vi "Get Table Configuration.vi"(8 "error in (no error)":errorcluster, 11 "Basic Table in":refnum<class "Basic Table.lvclass">) -> (0 "error out":errorcluster, 2 "Table Configuration":refnum<class "Table Configuration Interface.lvclass">, 3 "Basic Table out":refnum<class "Basic Table.lvclass">)   [LabVIEW 2020, in "Table.lvlib" / "Basic Table.lvclass"]
uses:
  Basic Table.lvclass
  Table Configuration Interface/Table Configuration Interface.lvclass
  Basic Table.lvclass/Basic Table.ctl
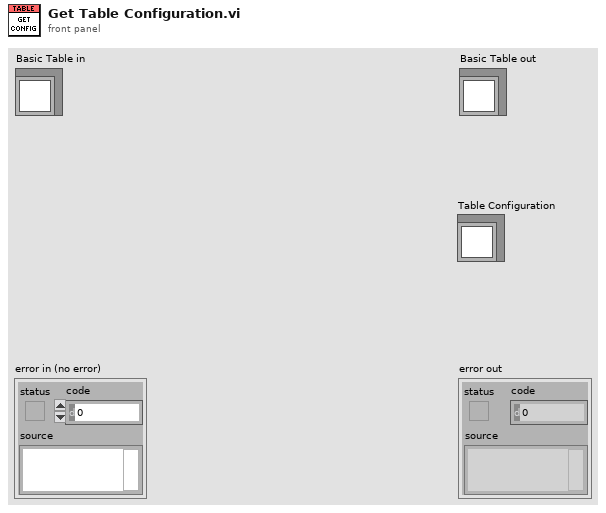
[diagram p1: front panel]
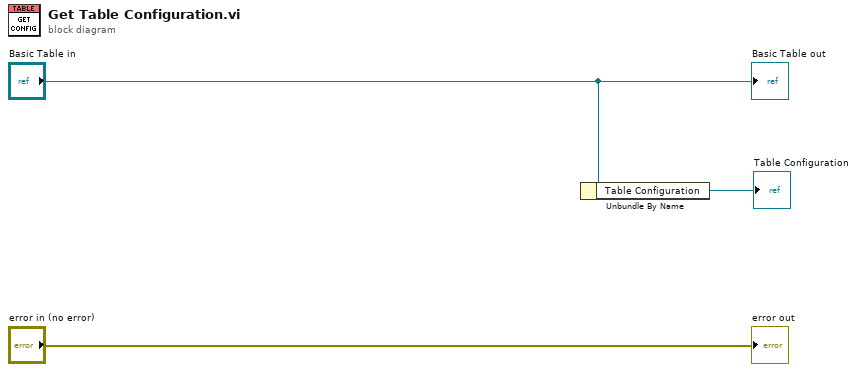
[diagram p0: block diagram]
diagram:
  n1 = Unbundle By Name("Basic Table in") -> ("Table Configuration"=→"Table Configuration":refnum<class "Table Configuration Interface.lvclass">)
  "error out" <- "error in (no error)"
  "Basic Table out" <- "Basic Table in"
